vi "Push_Data_via_Public_Server.vi"(2 "Archive File?":bool[](array[boolean]), 4 "Path of Files relative to EnFlo Data Root":path[](array[path])) -> (0 "error out":errorcluster, 1 "Problem Files":path[](array[path]))   [LabVIEW 2016]
uses:
  Anemometry/Anemometry Sub Vis/Globals/Constants_global.vi
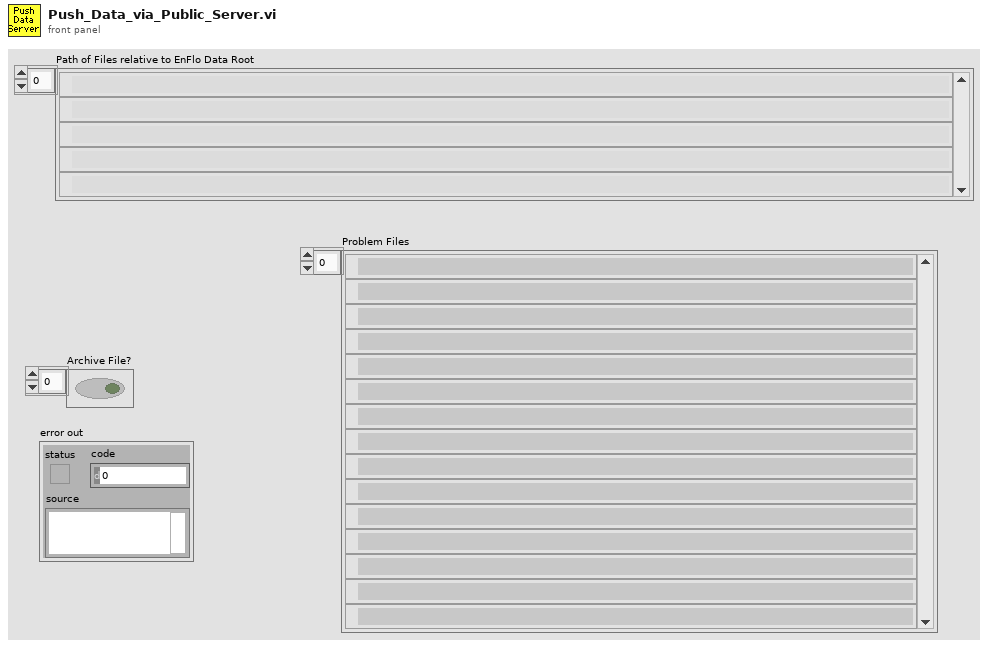
[diagram p1: front panel]
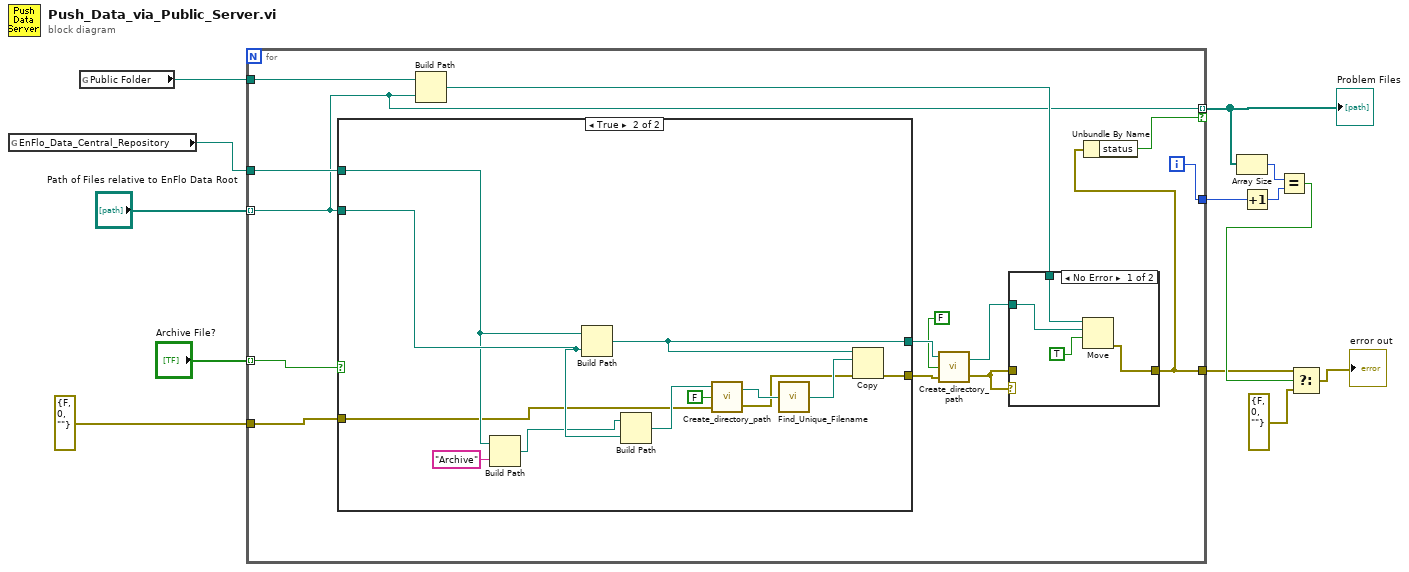
[diagram p0: block diagram]
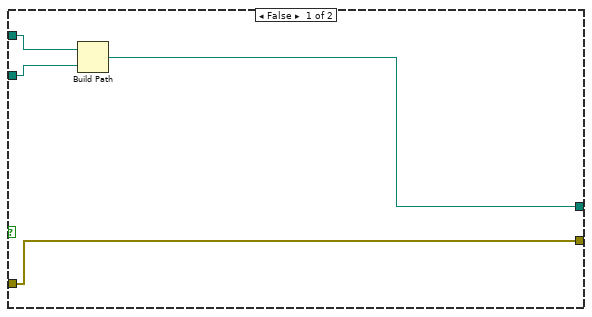
[diagram p2: hidden frame]
diagram:
  n1 = global read "Constants_global.vi" "EnFlo_Data_Central_Repository"() -> (w13:path)
  n2 = global read "Constants_global.vi" "Public Folder"() -> (w9:path)
  n3 = for {
    tunnel: [w16] -> w3
    tunnel: w13 -> [w27]
    tunnel: "Path of Files relative to EnFlo Data Root" -> [w17] mode=indexing
    tunnel: w9 -> [w22]
    tunnel: errorcluster {"status"=FALSE, "code"=0, "source"=""} ("error out") -> [w20]
    tunnel: "Archive File?" -> [w19] mode=indexing
    tunnel: [w17] -> w8 mode=indexing if=w15
    tunnel: [w14] -> w7
    i -> [w14]
    n4 = case shown="True" w19 {
      tunnel: w27 -> [w31 w37]
      tunnel: w17 -> [w30 w39]
      tunnel: [w28 w35] -> w26
      tunnel: w20 -> [w28 w34]
      tunnel: [w29 w33] -> w24
      frame False {
        n5 = Build Path(base path=w31, name or relative path=w30) -> (appended path=w29:path)
      }
      frame True {
        n6 = Build Path(base path=w37, name or relative path="Archive") -> (appended path=w36:path)
        n7 = Build Path(base path=w37, name or relative path=w39) -> (appended path=w33:path)
        n8 = Build Path(base path=w36, name or relative path=w39) -> (appended path=w42:path)
        n9 = call "Create_directory_path.vi"("error in (no error)"=w34, "Dialog Box"=FALSE, "Path name"=w42) -> ("error out"=w40:errorcluster, "Path name Out"=w41:path)
        n10 = call "Find_Unique_Filename.vi"("Path In"=w41) -> ("Unique Path Out"=w43:path)  [unwired: 2 in]
        n11 = Copy(8:w40, 10:w43, 11:w33) -> (0:w35:errorcluster)  [unwired: 2 in, 2 out]
      }
    }
    n12 = Build Path(base path=w22, name or relative path=w17) -> (appended path=w21:path)
    n13 = call "Create_directory_path.vi"("error in (no error)"=w26, "Dialog Box"=FALSE, "Path name"=w24) -> ("error out"=w25:errorcluster, "Path name Out"=w23:path)
    n14 = case shown="No Error" w25 {
      tunnel: [w45 w48] -> w16
      tunnel: w23 -> [w47 _]
      tunnel: w25 -> [_ w48]
      tunnel: w21 -> [w46 _]
      frame No Error {
        n15 = Move(source path=w46, 9:TRUE ("overwrite (F)"), 10:w47) -> (error out=w45:errorcluster)  [unwired: 2 in, 2 out]
      }
      frame Error {
      }
    }
    n16 = Unbundle By Name(w16) -> ("status"=w15:bool)
  }
  "Problem Files" <- w8
  n17 = Array Size(array=w8) -> (size(s)=w6:i32)
  n18 = Increment(x=w7) -> (x+1=w5:i32)
  n19 = Equal?(x=w6, y=w5) -> (x = y?=w4:bool)
  n20 = Select(t=w3, s=w4, f=errorcluster {"status"=FALSE, "code"=0, "source"=""} ("error out")) -> (s? t:f=→"error out":errorcluster)
